vi "Generator.Create Reference Waveforms.vi"(8 "error in (no error)":errorcluster, 10 "reset phase":bool, 11 "Lockin.DAQ in":refnum<class "Instrument.DAQ.lvclass">) -> (0 "error out":errorcluster, 1 "Y":waveform(dbl)[](array[waveform]), 2 "X":waveform(dbl)[](array[waveform]), 3 "Lockin.DAQ out":refnum<class "Instrument.DAQ.lvclass">)   [LabVIEW 2019, in "Instrument.DAQ.lvclass"]
uses:
  Instrument.DAQ.lvclass
  Typedefs/REF.Channel--Cluster--Array.ctl
  Typedefs/REF.Channel--Cluster.ctl
  Instrument.DAQ.lvclass/Instrument.DAQ.ctl
  <vilib>/measure/NI_MABase.lvlib
  Typedefs/DAQ.Sampling.Sampling--Cluster.ctl
panel:
  in  "Configuration.Channels: REF":T1 {"Roll-Off" min=1; "TC" min=0.0001 format="%#_3p"; "Phase" format="%.3g"; "Frequency" min=0.0001 max=10000.0 format="%.3g"; "Channel" min=1}
  in  "Update Graph?":bool
  out "Waveform Graph":waveform(dbl)[](graph)
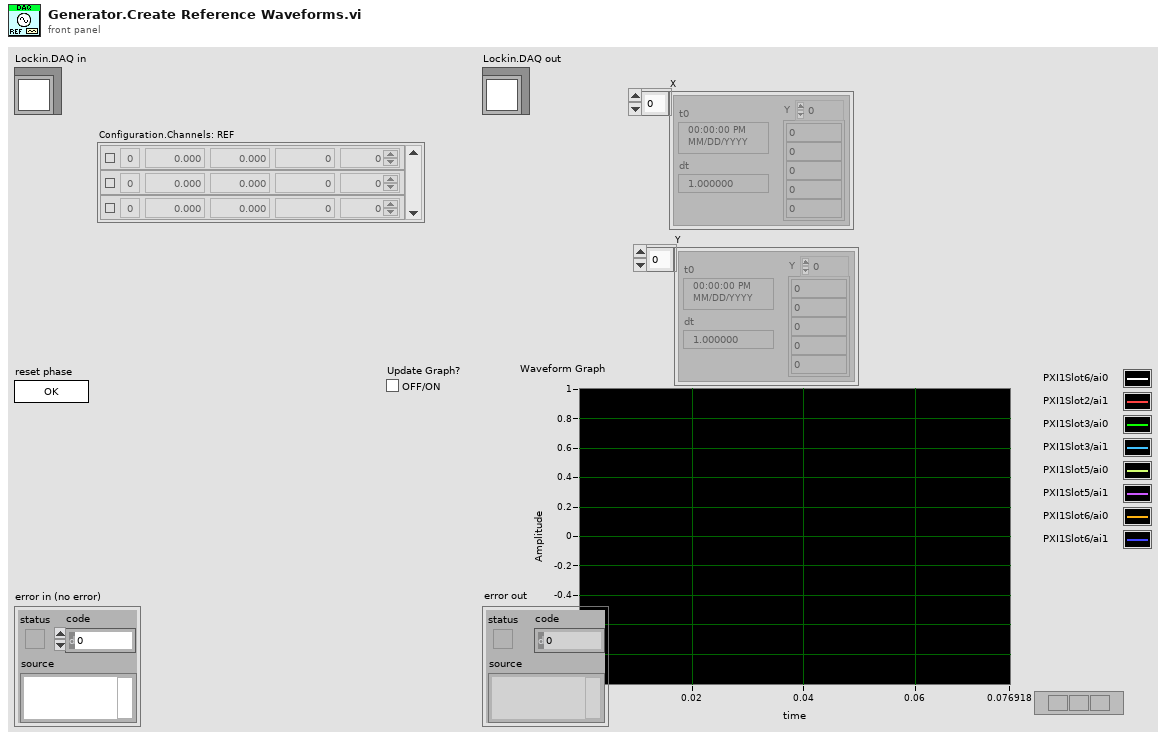
[diagram p1: front panel]
types:
  T1 = typedef "Instrument.DAQ.lvclass/REF.Channel--Cluster--Array.ctl" = T2[]
  T2 = typedef "Instrument.DAQ.lvclass/REF.Channel--Cluster.ctl" = cluster{"Enable?":bool, "Channel":i32, "Frequency":dbl, "Phase":dbl, "TC":dbl, "Roll-Off":i32}
  T3 = typedef "Instrument.DAQ.lvclass/DAQ.Sampling.Sampling--Cluster.ctl" = cluster{"Fs":dbl, "#s":i32}
  T4 = enum16{"Sine Wave", "Triangle Wave", "Square Wave", "Sawtooth Wave"}
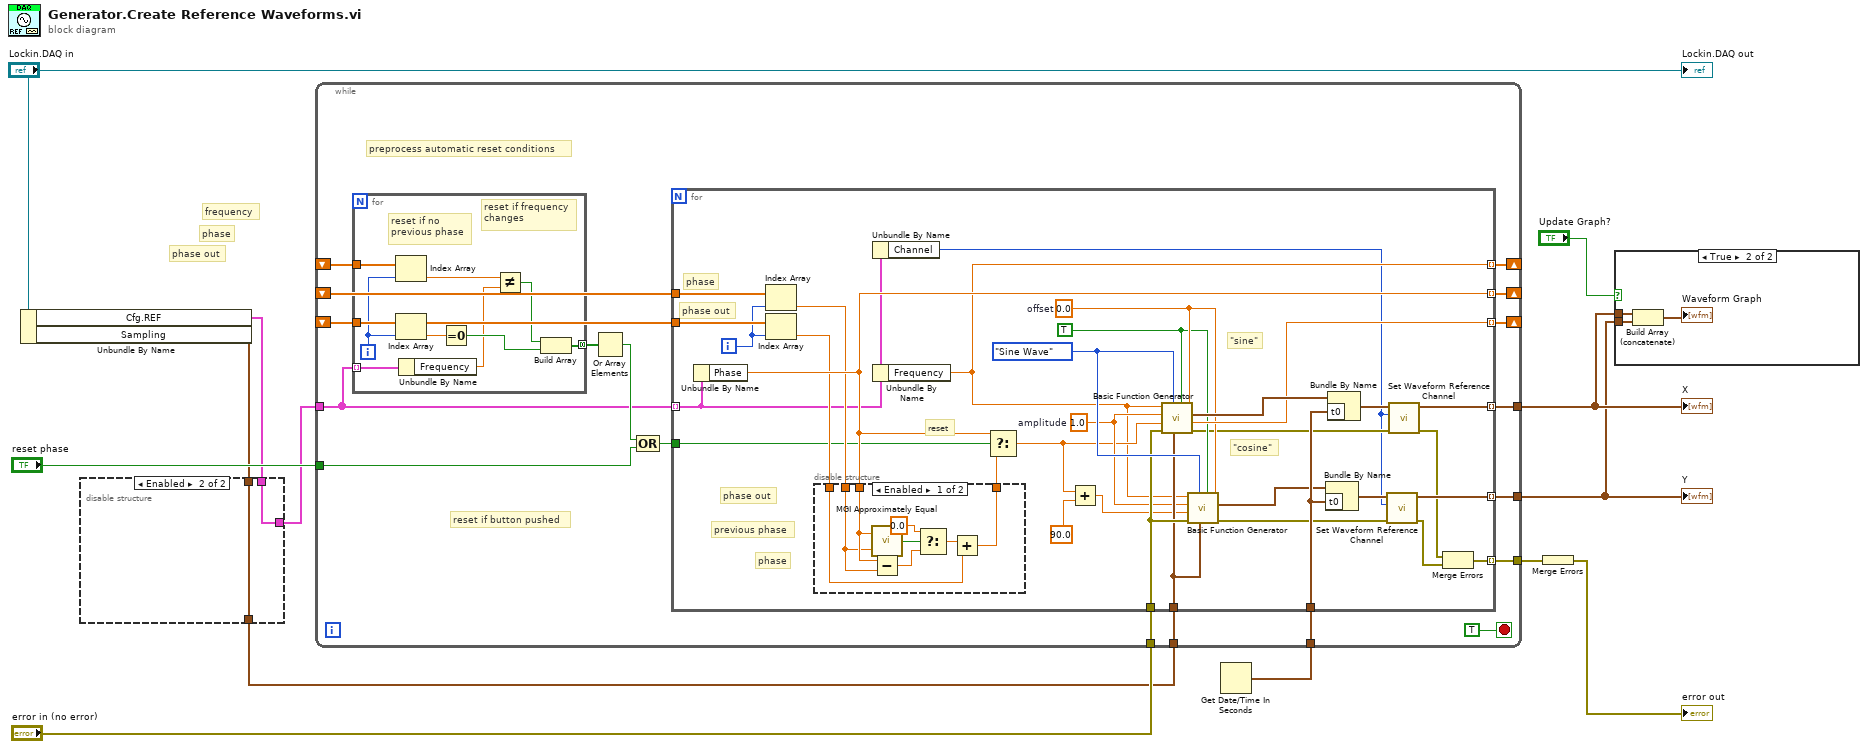
[diagram p0: block diagram]
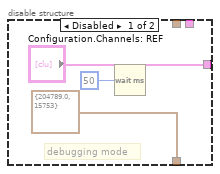
[diagram p2: hidden frame]
diagram:
  # "phase out"
  # "phase"
  # "frequency"
  n1 = Unbundle By Name("Lockin.DAQ in") -> ("Cfg.REF"=w4:T1, "Sampling"=w5:T3)
  n2 = disable-structure shown="Enabled" {
    disable-tunnel: [T3 {"Fs"=204789.0, "#s"=15753} ("Configuration.DAQ.sampling") w18] -> w6
    disable-tunnel: w5 -> [_ w18]
    disable-tunnel: ["Configuration.Channels: REF" w17] -> w3
    disable-tunnel: w4 -> [_ w17]
    frame Disabled {
      # "debugging mode"
      n3 = Wait (ms)(milliseconds to wait=u32 50) -> ()  [unwired: 1 out]
    }
    frame Enabled {
    }
  }
  n4 = Get Date/Time In Seconds() -> (seconds since 1Jan1904=w11:timestamp)
  n5 = while {
    tunnel: w6 -> [w36]
    shift-right: [w34] -> _
    shift-left: _ -> [w28]
    tunnel: w11 -> [w33]
    tunnel: "reset phase" -> [w23]
    tunnel: "error in (no error)" -> [w32]
    tunnel: w3 -> [w21]
    shift-right: [w31] -> _
    shift-left: _ -> [w26]
    shift-right: [w30] -> _
    shift-left: _ -> [w27]
    tunnel: [w29] -> w8
    tunnel: [w20] -> w2
    tunnel: [w19] -> w1
    stop <- TRUE stop-if-true
    # "preprocess automatic reset conditions"
    # "reset if button pushed"
    n6 = for {
      tunnel: w21 -> [w38] mode=indexing
      tunnel: w28 -> [w45]
      tunnel: w26 -> [w44]
      tunnel: [w39] -> w25 mode=concatenating
      i -> [w46]
      # "reset if frequency\nchanges"
      # "reset if no\nprevious phase"
      n7 = Index Array(array=w44, index=w46) -> (element=w42:dbl)
      n8 = Index Array(array=w45, index=w46) -> (element=w43:dbl)
      n9 = Unbundle By Name(w38) -> ("Frequency"=w37:dbl)
      n10 = Equal To 0?(x=w43) -> (x = 0?=w40:bool)
      n11 = Not Equal?(x=w42, y=w37) -> (x != y?=w41:bool)
      n12 = Build Array(w41, w40) -> (w39:bool[])
    }
    n13 = Or Array Elements(Boolean array=w25) -> (logical OR=w24:bool)
    n14 = Compound Arithmetic op=OR(w24, w23) -> (w22:bool)
    n15 = for {
      tunnel: w36 -> [w71]
      tunnel: [w77] -> w34 mode=indexing
      tunnel: w33 -> [w76]
      tunnel: w32 -> [w72]
      tunnel: w21 -> [w49] mode=indexing
      tunnel: w28 -> [w68]
      tunnel: [w59] -> w31 mode=indexing
      tunnel: [w64] -> w30 mode=indexing
      tunnel: w22 -> [w60]
      tunnel: w27 -> [w67]
      tunnel: [w66] -> w29 mode=indexing
      tunnel: [w57] -> w20 mode=indexing
      tunnel: [w55] -> w19 mode=indexing
      i -> [w54]
      w69 = TRUE ("reset signal")
      w73 = 0.0  # offset
      w74 = T4."Sine Wave" ("signal type")
      w70 = 1.0  # amplitude
      # "phase out"
      # "phase"
      # "previous phase"
      # "phase"
      # "phase out"
      # "reset"
      # "\"cosine\""
      # "\"sine\""
      n16 = Unbundle By Name(w49) -> ("Phase"=w64:dbl)
      n17 = Index Array(array=w67, index=w54) -> (element=w63:dbl)
      n18 = Index Array(array=w68, index=w54) -> (element=w61:dbl)
      n19 = disable-structure shown="Enabled" {
        disable-tunnel: w64 -> [w86 _]
        disable-tunnel: w63 -> [w85 _]
        disable-tunnel: w61 -> [w80 w88]
        disable-tunnel: [w83 w88] -> w62
        frame Enabled {
          n20 = call <userlib>:"MGI Approximately Equal.vi"("Numeric 2"=w85, "Numeric 1"=w86) -> ("approx = ?"=w84:bool)
          n21 = Subtract(x=w86, y=w85) -> (x-y=w82:dbl)
          n22 = Select(t=0.0, s=w84, f=w82) -> (s? t:f=w81:dbl)
          n23 = Add(x=w81, y=w80) -> (x+y=w83:dbl)
        }
        frame Disabled {
        }
      }
      n24 = Unbundle By Name(w49) -> ("Channel"=w48:i32)
      n25 = Unbundle By Name(w49) -> ("Frequency"=w59:dbl)
      n26 = Select(t=w64, s=w60, f=w62) -> (s? t:f=w65:dbl)
      n27 = Add(x=w65, y=90.0) -> (x+y=w47:dbl)
      n28 = call <vilib>:"Basic Function Generator.vi"("offset"=w73, "reset signal"=w69, "sampling info"=w71, "signal type"=w74, "error in (no error)"=w72, "phase"=w65, "amplitude"=w70, "frequency"=w59) -> ("error out"=w53:errorcluster, "phase out"=w77:dbl, "signal out"=w79:waveform(dbl))  [unwired: 1 in]
      n29 = call <vilib>:"Basic Function Generator.vi"("offset"=w73, "reset signal"=w69, "sampling info"=w71, "signal type"=w74, "error in (no error)"=w72, "phase"=w47, "amplitude"=w70, "frequency"=w59) -> ("error out"=w52:errorcluster, "signal out"=w75:waveform(dbl))  [unwired: 1 in, 1 out]
      n30 = Bundle By Name(cluster=w75, "t0"=w76) -> (w56:waveform(dbl))
      n31 = Bundle By Name(cluster=w79, "t0"=w76) -> (w58:waveform(dbl))
      n32 = call "Set Waveform Reference Channel.vi"("error in (no error)"=w52, "Reference Ch"=w48, "Waveform in"=w56) -> ("error out"=w51:errorcluster, "Waveform out"=w55:waveform(dbl))  [unwired: 7 in]
      n33 = call "Set Waveform Reference Channel.vi"("error in (no error)"=w53, "Reference Ch"=w48, "Waveform in"=w58) -> ("error out"=w50:errorcluster, "Waveform out"=w57:waveform(dbl))  [unwired: 7 in]
      n34 = Merge Errors(w50, w51) -> (w66:errorcluster)
    }
  }
  "X" <- w2
  "Y" <- w1
  n35 = Merge Errors(w8) -> (→"error out":errorcluster)
  n36 = case shown="True" "Update Graph?" {
    tunnel: w2 -> [_ w90]
    tunnel: w1 -> [_ w89]
    frame False {
    }
    frame True {
      n37 = Build Array (concatenate)(w90, w89) -> (→"Waveform Graph":waveform(dbl)[])
    }
  }
  "Lockin.DAQ out" <- "Lockin.DAQ in"
